vi "Get Multiplexer.vi"(11 "CANopen Message in":refnum<class "CANopen Message.lvclass">) -> (2 "Multiplexer":T1 {"Sub-Index" format="%.0x"; "Index" format="%04x"}, 3 "CANopen Message out":refnum<class "CANopen Message.lvclass">)   [LabVIEW 2024, in "CANopen Master.lvlib" / "CANopen Message.lvclass"]
uses:
  CANopen Message.lvclass
  CANopen Message.lvclass/CANopen Message.ctl
  CANopen/Multiplexor.ctl
  CANopen Master.lvlib
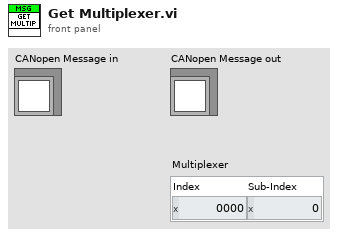
[diagram p1: front panel]
types:
  T1 = typedef "CANopen Master.lvlib/Multiplexor.ctl" = cluster{"Index":u16, "Sub-Index":i16}
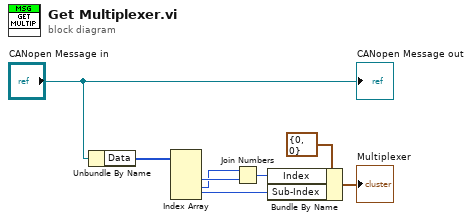
[diagram p0: block diagram]
diagram:
  n1 = Unbundle By Name("CANopen Message in") -> ("Data"=w7:u8[])
  n2 = Index Array(array=w7) -> (element #2=w6:u8, element #3=w5:u8, element #4=w2:u8)  [unwired: 4 in, 1 out]
  n3 = Join Numbers(hi=w5, lo=w6) -> ((hi.lo)=w3:u16)
  n4 = Bundle By Name(cluster=T1 {"Index"=0, "Sub-Index"=0} ("Multiplexer"), "Index"=w3, "Sub-Index"=w2) -> (→"Multiplexer":T1)
  "CANopen Message out" <- "CANopen Message in"
